vi "S4GUI.vi"(7 "Tab ObsEng":enum32{"Obs", "CCD modes", "Eng"}(tab)) -> ()   [LabVIEW 2018] (continued)
            n1626 = call-dynamic "Read Channel.vi"("error in (no error)"=w3103, "Acquisition in"=w3105) -> ("error out"=w3098:errorcluster, "Channel.lvclass"=w3100:refnum<class "Channel.lvclass">, "Acquisition out"=w3104:refnum<class "Acquisition.lvclass">)  [unwired: 7 in]
            n1627 = call "Write section_name.vi"("error in (no error)"=w3098, "section_name"="CCD_ACS1", "Channel in"=w3100) -> ("error out"=w3097:errorcluster, "Channel out"=w3099:refnum<class "Channel.lvclass">)  [unwired: 7 in]
            n1628 = call-dynamic "save config.vi"("error in (no error)"=w3097, "file config"=w3051, "Channel in"=w3099) -> ("error out"=w3049:errorcluster, "Channel out"=w3050:refnum<class "Channel.lvclass">)  [unwired: 7 in]
            n1629 = call-dynamic "Write Channel.vi"("error in (no error)"=w3049, "Channel.lvclass"=w3050, "Acquisition in"=w3104) -> ("error out"=w3102:errorcluster, "Acquisition out"=w3101:refnum<class "Acquisition.lvclass">)  [unwired: 7 in]
            n1630 = call-dynamic "Write AcquisitionA.vi"("error in (no error)"=w3102, "Acquisition.lvclass"=w3101, "S4ACS_GUI in"=w3106) -> ("error out"=w3062:errorcluster, "S4ACS_GUI out"=w3061:refnum<class "S4GUI.lvclass">)  [unwired: 7 in]
            n1631 = call "Read AcquisitionB.vi"("error in (no error)"=w3062, "S4ACS_GUI in"=w3061) -> ("error out"=w3088:errorcluster, "Acquisition.lvclass"=w3086:refnum<class "Acquisition.lvclass">, "S4ACS_GUI out"=w3085:refnum<class "S4GUI.lvclass">)  [unwired: 7 in]
            n1632 = call-dynamic "Read Channel.vi"("error in (no error)"=w3088, "Acquisition in"=w3086) -> ("error out"=w3093:errorcluster, "Channel.lvclass"=w3091:refnum<class "Channel.lvclass">, "Acquisition out"=w3087:refnum<class "Acquisition.lvclass">)  [unwired: 7 in]
            n1633 = call "Write section_name.vi"("error in (no error)"=w3093, "section_name"="CCD_ACS2", "Channel in"=w3091) -> ("error out"=w3094:errorcluster, "Channel out"=w3092:refnum<class "Channel.lvclass">)  [unwired: 7 in]
            n1634 = call-dynamic "save config.vi"("error in (no error)"=w3094, "file config"=w3051, "Channel in"=w3092) -> ("error out"=w3043:errorcluster, "Channel out"=w3044:refnum<class "Channel.lvclass">)  [unwired: 7 in]
            n1635 = call-dynamic "Write Channel.vi"("error in (no error)"=w3043, "Channel.lvclass"=w3044, "Acquisition in"=w3087) -> ("error out"=w3089:errorcluster, "Acquisition out"=w3090:refnum<class "Acquisition.lvclass">)  [unwired: 7 in]
            n1636 = call "Write AcquisitionB.vi"("error in (no error)"=w3089, "Acquisition.lvclass"=w3090, "S4ACS_GUI in"=w3085) -> ("error out"=w3060:errorcluster, "S4ACS_GUI out"=w3059:refnum<class "S4GUI.lvclass">)  [unwired: 7 in]
            n1637 = call-dynamic "Read AcquisitionC.vi"("error in (no error)"=w3060, "S4ACS_GUI in"=w3059) -> ("error out"=w3081:errorcluster, "Acquisition.lvclass"=w3083:refnum<class "Acquisition.lvclass">, "S4ACS_GUI out"=w3084:refnum<class "S4GUI.lvclass">)  [unwired: 7 in]
            n1638 = call-dynamic "Read Channel.vi"("error in (no error)"=w3081, "Acquisition in"=w3083) -> ("error out"=w3076:errorcluster, "Channel.lvclass"=w3078:refnum<class "Channel.lvclass">, "Acquisition out"=w3082:refnum<class "Acquisition.lvclass">)  [unwired: 7 in]
            n1639 = call "Write section_name.vi"("error in (no error)"=w3076, "section_name"="CCD_ACS3", "Channel in"=w3078) -> ("error out"=w3075:errorcluster, "Channel out"=w3077:refnum<class "Channel.lvclass">)  [unwired: 7 in]
            n1640 = call-dynamic "save config.vi"("error in (no error)"=w3075, "file config"=w3051, "Channel in"=w3077) -> ("error out"=w3045:errorcluster, "Channel out"=w3046:refnum<class "Channel.lvclass">)  [unwired: 7 in]
            n1641 = call-dynamic "Write Channel.vi"("error in (no error)"=w3045, "Channel.lvclass"=w3046, "Acquisition in"=w3082) -> ("error out"=w3080:errorcluster, "Acquisition out"=w3079:refnum<class "Acquisition.lvclass">)  [unwired: 7 in]
            n1642 = call-dynamic "Write AcquisitionC.vi"("error in (no error)"=w3080, "Acquisition.lvclass"=w3079, "S4ACS_GUI in"=w3084) -> ("error out"=w3058:errorcluster, "S4ACS_GUI out"=w3057:refnum<class "S4GUI.lvclass">)  [unwired: 7 in]
            n1643 = call-dynamic "Read AcquisitionD.vi"("error in (no error)"=w3058, "S4ACS_GUI in"=w3057) -> ("error out"=w3066:errorcluster, "Acquisition.lvclass"=w3064:refnum<class "Acquisition.lvclass">, "S4ACS_GUI out"=w3063:refnum<class "S4GUI.lvclass">)  [unwired: 7 in]
            n1644 = call-dynamic "Read Channel.vi"("error in (no error)"=w3066, "Acquisition in"=w3064) -> ("error out"=w3071:errorcluster, "Channel.lvclass"=w3069:refnum<class "Channel.lvclass">, "Acquisition out"=w3065:refnum<class "Acquisition.lvclass">)  [unwired: 7 in]
            n1645 = call "Write section_name.vi"("error in (no error)"=w3071, "section_name"="CCD_ACS4", "Channel in"=w3069) -> ("error out"=w3072:errorcluster, "Channel out"=w3070:refnum<class "Channel.lvclass">)  [unwired: 7 in]
            n1646 = call-dynamic "save config.vi"("error in (no error)"=w3072, "file config"=w3051, "Channel in"=w3070) -> ("error out"=w3047:errorcluster, "Channel out"=w3048:refnum<class "Channel.lvclass">)  [unwired: 7 in]
            n1647 = call-dynamic "Write Channel.vi"("error in (no error)"=w3047, "Channel.lvclass"=w3048, "Acquisition in"=w3065) -> ("error out"=w3067:errorcluster, "Acquisition out"=w3068:refnum<class "Acquisition.lvclass">)  [unwired: 7 in]
            n1648 = call-dynamic "Write AcquisitionD.vi"("error in (no error)"=w3067, "Acquisition.lvclass"=w3068, "S4ACS_GUI in"=w3063) -> ("error out"=w3054:errorcluster, "S4ACS_GUI out"=w3056:refnum<class "S4GUI.lvclass">)  [unwired: 7 in]
            n1649 = call "Write cfg file.vi"("error in (no error)"=w3054, "cfg file"=w3051, "S4ACS_GUI in"=w3056) -> ("error out"=w3053:errorcluster, "S4ACS_GUI out"=w3055:refnum<class "S4GUI.lvclass">)  [unwired: 7 in]
          }
          frame True {
          }
        }
      }
      event "Load Default Button": Value Change {
        w3130 = "default.cfg" ("cfg file name")
        n1650 = event-data() -> ()  [unwired: 1 in, 6 out]
        n1651 = call-dynamic "Read AcquisitionA.vi"("error in (no error)"=w3220, "S4ACS_GUI in"=w3221) -> ("error out"=w3216:errorcluster, "Acquisition.lvclass"=w3218:refnum<class "Acquisition.lvclass">, "S4ACS_GUI out"=w3219:refnum<class "S4GUI.lvclass">)  [unwired: 7 in]
        n1652 = call-dynamic "Read Channel.vi"("error in (no error)"=w3216, "Acquisition in"=w3218) -> ("error out"=w3203:errorcluster, "Channel.lvclass"=w3205:refnum<class "Channel.lvclass">, "Acquisition out"=w3217:refnum<class "Acquisition.lvclass">)  [unwired: 7 in]
        n1653 = call "Write section_name.vi"("error in (no error)"=w3203, "section_name"="CCD_ACS1", "Channel in"=w3205) -> ("error out"=w3202:errorcluster, "Channel out"=w3204:refnum<class "Channel.lvclass">)  [unwired: 7 in]
        n1654 = call-dynamic "load config.vi"("error in (no error)"=w3202, "cfg file name"=w3130, "Channel in"=w3204) -> ("error out"=w3127:errorcluster, "Channel out"=w3129:refnum<class "Channel.lvclass">)  [unwired: 7 in]
        n1655 = call-dynamic "save config.vi"("error in (no error)"=w3127, "file config"="lastsaved.cfg", "Channel in"=w3129) -> ("error out"=w3126:errorcluster, "Channel out"=w3128:refnum<class "Channel.lvclass">)  [unwired: 7 in]
        n1656 = call-dynamic "Read State Machine.vi"("error in (no error)"=w3126, "Device in"=w3128) -> ("error out"=w3212:errorcluster, "State Machine.lvclass"=w3214:refnum<class "State Machine.lvclass">, "Device out"=w3215:refnum<class "Channel.lvclass">)  [unwired: 7 in]
        n1657 = call-dynamic "Write State.vi"("error in (no error)"=w3212, "State"=60, "State Machine in"=w3214) -> ("error out"=w3211:errorcluster, "State Machine out"=w3213:refnum<class "State Machine.lvclass">)  [unwired: 7 in]
        n1658 = call-dynamic "Write State Machine.vi"("error in (no error)"=w3211, "State Machine.lvclass"=w3213, "Device in"=w3215) -> ("error out"=w3208:errorcluster, "Device out"=w3209:refnum<class "Channel.lvclass">)  [unwired: 7 in]
        n1659 = call-dynamic "Write Channel.vi"("error in (no error)"=w3208, "Channel.lvclass"=w3209, "Acquisition in"=w3217) -> ("error out"=w3207:errorcluster, "Acquisition out"=w3206:refnum<class "Acquisition.lvclass">)  [unwired: 7 in]
        n1660 = call-dynamic "Write AcquisitionA.vi"("error in (no error)"=w3207, "Acquisition.lvclass"=w3206, "S4ACS_GUI in"=w3219) -> ("error out"=w3140:errorcluster, "S4ACS_GUI out"=w3139:refnum<class "S4GUI.lvclass">)  [unwired: 7 in]
        n1661 = call "Read AcquisitionB.vi"("error in (no error)"=w3140, "S4ACS_GUI in"=w3139) -> ("error out"=w3184:errorcluster, "Acquisition.lvclass"=w3182:refnum<class "Acquisition.lvclass">, "S4ACS_GUI out"=w3181:refnum<class "S4GUI.lvclass">)  [unwired: 7 in]
        n1662 = call-dynamic "Read Channel.vi"("error in (no error)"=w3184, "Acquisition in"=w3182) -> ("error out"=w3198:errorcluster, "Channel.lvclass"=w3196:refnum<class "Channel.lvclass">, "Acquisition out"=w3183:refnum<class "Acquisition.lvclass">)  [unwired: 7 in]
        n1663 = call "Write section_name.vi"("error in (no error)"=w3198, "section_name"="CCD_ACS2", "Channel in"=w3196) -> ("error out"=w3199:errorcluster, "Channel out"=w3197:refnum<class "Channel.lvclass">)  [unwired: 7 in]
        n1664 = call-dynamic "load config.vi"("error in (no error)"=w3199, "cfg file name"="default.cfg", "Channel in"=w3197) -> ("error out"=w3123:errorcluster, "Channel out"=w3121:refnum<class "Channel.lvclass">)  [unwired: 7 in]
        n1665 = call-dynamic "save config.vi"("error in (no error)"=w3123, "file config"="lastsaved.cfg", "Channel in"=w3121) -> ("error out"=w3122:errorcluster, "Channel out"=w3120:refnum<class "Channel.lvclass">)  [unwired: 7 in]
        n1666 = call-dynamic "Read State Machine.vi"("error in (no error)"=w3122, "Device in"=w3120) -> ("error out"=w3188:errorcluster, "State Machine.lvclass"=w3186:refnum<class "State Machine.lvclass">, "Device out"=w3185:refnum<class "Channel.lvclass">)  [unwired: 7 in]
        n1667 = call-dynamic "Write State.vi"("error in (no error)"=w3188, "State"=60, "State Machine in"=w3186) -> ("error out"=w3189:errorcluster, "State Machine out"=w3187:refnum<class "State Machine.lvclass">)  [unwired: 7 in]
        n1668 = call-dynamic "Write State Machine.vi"("error in (no error)"=w3189, "State Machine.lvclass"=w3187, "Device in"=w3185) -> ("error out"=w3192:errorcluster, "Device out"=w3191:refnum<class "Channel.lvclass">)  [unwired: 7 in]
        n1669 = call-dynamic "Write Channel.vi"("error in (no error)"=w3192, "Channel.lvclass"=w3191, "Acquisition in"=w3183) -> ("error out"=w3193:errorcluster, "Acquisition out"=w3194:refnum<class "Acquisition.lvclass">)  [unwired: 7 in]
        n1670 = call "Write AcquisitionB.vi"("error in (no error)"=w3193, "Acquisition.lvclass"=w3194, "S4ACS_GUI in"=w3181) -> ("error out"=w3138:errorcluster, "S4ACS_GUI out"=w3137:refnum<class "S4GUI.lvclass">)  [unwired: 7 in]
        n1671 = call-dynamic "Read AcquisitionC.vi"("error in (no error)"=w3138, "S4ACS_GUI in"=w3137) -> ("error out"=w3177:errorcluster, "Acquisition.lvclass"=w3179:refnum<class "Acquisition.lvclass">, "S4ACS_GUI out"=w3180:refnum<class "S4GUI.lvclass">)  [unwired: 7 in]
        n1672 = call-dynamic "Read Channel.vi"("error in (no error)"=w3177, "Acquisition in"=w3179) -> ("error out"=w3163:errorcluster, "Channel.lvclass"=w3165:refnum<class "Channel.lvclass">, "Acquisition out"=w3178:refnum<class "Acquisition.lvclass">)  [unwired: 7 in]
        n1673 = call "Write section_name.vi"("error in (no error)"=w3163, "section_name"="CCD_ACS3", "Channel in"=w3165) -> ("error out"=w3162:errorcluster, "Channel out"=w3164:refnum<class "Channel.lvclass">)  [unwired: 7 in]
        n1674 = call-dynamic "load config.vi"("error in (no error)"=w3162, "cfg file name"="default.cfg", "Channel in"=w3164) -> ("error out"=w3117:errorcluster, "Channel out"=w3118:refnum<class "Channel.lvclass">)  [unwired: 7 in]
        n1675 = call-dynamic "save config.vi"("error in (no error)"=w3117, "file config"="lastsaved.cfg", "Channel in"=w3118) -> ("error out"=w3115:errorcluster, "Channel out"=w3116:refnum<class "Channel.lvclass">)  [unwired: 7 in]
        n1676 = call-dynamic "Read State Machine.vi"("error in (no error)"=w3115, "Device in"=w3116) -> ("error out"=w3173:errorcluster, "State Machine.lvclass"=w3175:refnum<class "State Machine.lvclass">, "Device out"=w3176:refnum<class "Channel.lvclass">)  [unwired: 7 in]
        n1677 = call-dynamic "Write State.vi"("error in (no error)"=w3173, "State"=60, "State Machine in"=w3175) -> ("error out"=w3172:errorcluster, "State Machine out"=w3174:refnum<class "State Machine.lvclass">)  [unwired: 7 in]
        n1678 = call-dynamic "Write State Machine.vi"("error in (no error)"=w3172, "State Machine.lvclass"=w3174, "Device in"=w3176) -> ("error out"=w3169:errorcluster, "Device out"=w3170:refnum<class "Channel.lvclass">)  [unwired: 7 in]
        n1679 = call-dynamic "Write Channel.vi"("error in (no error)"=w3169, "Channel.lvclass"=w3170, "Acquisition in"=w3178) -> ("error out"=w3168:errorcluster, "Acquisition out"=w3167:refnum<class "Acquisition.lvclass">)  [unwired: 7 in]
        n1680 = call-dynamic "Write AcquisitionC.vi"("error in (no error)"=w3168, "Acquisition.lvclass"=w3167, "S4ACS_GUI in"=w3180) -> ("error out"=w3136:errorcluster, "S4ACS_GUI out"=w3135:refnum<class "S4GUI.lvclass">)  [unwired: 7 in]
        n1681 = call-dynamic "Read AcquisitionD.vi"("error in (no error)"=w3136, "S4ACS_GUI in"=w3135) -> ("error out"=w3144:errorcluster, "Acquisition.lvclass"=w3142:refnum<class "Acquisition.lvclass">, "S4ACS_GUI out"=w3141:refnum<class "S4GUI.lvclass">)  [unwired: 7 in]
        n1682 = call-dynamic "Read Channel.vi"("error in (no error)"=w3144, "Acquisition in"=w3142) -> ("error out"=w3158:errorcluster, "Channel.lvclass"=w3156:refnum<class "Channel.lvclass">, "Acquisition out"=w3143:refnum<class "Acquisition.lvclass">)  [unwired: 7 in]
        n1683 = call "Write section_name.vi"("error in (no error)"=w3158, "section_name"="CCD_ACS4", "Channel in"=w3156) -> ("error out"=w3159:errorcluster, "Channel out"=w3157:refnum<class "Channel.lvclass">)  [unwired: 7 in]
        n1684 = call-dynamic "load config.vi"("error in (no error)"=w3159, "cfg file name"="default.cfg", "Channel in"=w3157) -> ("error out"=w3113:errorcluster, "Channel out"=w3112:refnum<class "Channel.lvclass">)  [unwired: 7 in]
        n1685 = call-dynamic "save config.vi"("error in (no error)"=w3113, "file config"="lastsaved.cfg", "Channel in"=w3112) -> ("error out"=w3110:errorcluster, "Channel out"=w3111:refnum<class "Channel.lvclass">)  [unwired: 7 in]
        n1686 = call-dynamic "Read State Machine.vi"("error in (no error)"=w3110, "Device in"=w3111) -> ("error out"=w3148:errorcluster, "State Machine.lvclass"=w3146:refnum<class "State Machine.lvclass">, "Device out"=w3145:refnum<class "Channel.lvclass">)  [unwired: 7 in]
        n1687 = call-dynamic "Write State.vi"("error in (no error)"=w3148, "State"=60, "State Machine in"=w3146) -> ("error out"=w3149:errorcluster, "State Machine out"=w3147:refnum<class "State Machine.lvclass">)  [unwired: 7 in]
        n1688 = call-dynamic "Write State Machine.vi"("error in (no error)"=w3149, "State Machine.lvclass"=w3147, "Device in"=w3145) -> ("error out"=w3152:errorcluster, "Device out"=w3151:refnum<class "Channel.lvclass">)  [unwired: 7 in]
        n1689 = call-dynamic "Write Channel.vi"("error in (no error)"=w3152, "Channel.lvclass"=w3151, "Acquisition in"=w3143) -> ("error out"=w3153:errorcluster, "Acquisition out"=w3154:refnum<class "Acquisition.lvclass">)  [unwired: 7 in]
        n1690 = call-dynamic "Write AcquisitionD.vi"("error in (no error)"=w3153, "Acquisition.lvclass"=w3154, "S4ACS_GUI in"=w3141) -> ("error out"=w3132:errorcluster, "S4ACS_GUI out"=w3134:refnum<class "S4GUI.lvclass">)  [unwired: 7 in]
        n1691 = call "Write cfg file.vi"("error in (no error)"=w3132, "cfg file"=w3130, "S4ACS_GUI in"=w3134) -> ("error out"=w3131:errorcluster, "S4ACS_GUI out"=w3133:refnum<class "S4GUI.lvclass">)  [unwired: 7 in]
      }
      event "Restore Default ch2": Value Change {
        n1692 = event-data() -> ()  [unwired: 1 in, 6 out]
        n1693 = call "Read AcquisitionB.vi"("error in (no error)"=w3252, "S4ACS_GUI in"=w3253) -> ("error out"=w3248:errorcluster, "Acquisition.lvclass"=w3250:refnum<class "Acquisition.lvclass">, "S4ACS_GUI out"=w3251:refnum<class "S4GUI.lvclass">)  [unwired: 7 in]
        n1694 = call-dynamic "Read Channel.vi"("error in (no error)"=w3248, "Acquisition in"=w3250) -> ("error out"=w3235:errorcluster, "Channel.lvclass"=w3237:refnum<class "Channel.lvclass">, "Acquisition out"=w3249:refnum<class "Acquisition.lvclass">)  [unwired: 7 in]
        n1695 = call "Write section_name.vi"("error in (no error)"=w3235, "section_name"="CCD_ACS2", "Channel in"=w3237) -> ("error out"=w3234:errorcluster, "Channel out"=w3236:refnum<class "Channel.lvclass">)  [unwired: 7 in]
        n1696 = call-dynamic "load config.vi"("error in (no error)"=w3234, "cfg file name"="default.cfg", "Channel in"=w3236) -> ("error out"=w3232:errorcluster, "Channel out"=w3233:refnum<class "Channel.lvclass">)  [unwired: 7 in]
        n1697 = call-dynamic "Read State Machine.vi"("error in (no error)"=w3232, "Device in"=w3233) -> ("error out"=w3244:errorcluster, "State Machine.lvclass"=w3246:refnum<class "State Machine.lvclass">, "Device out"=w3247:refnum<class "Channel.lvclass">)  [unwired: 7 in]
        n1698 = call-dynamic "Write State.vi"("error in (no error)"=w3244, "State"=60, "State Machine in"=w3246) -> ("error out"=w3243:errorcluster, "State Machine out"=w3245:refnum<class "State Machine.lvclass">)  [unwired: 7 in]
        n1699 = call-dynamic "Write State Machine.vi"("error in (no error)"=w3243, "State Machine.lvclass"=w3245, "Device in"=w3247) -> ("error out"=w3228:errorcluster, "Device out"=w3225:refnum<class "Channel.lvclass">)  [unwired: 7 in]
        n1700 = call "Write section_name.vi"("error in (no error)"=w3228, "section_name"="CCD_ACS2", "Channel in"=w3225) -> ("error out"=w3229:errorcluster, "Channel out"=w3224:refnum<class "Channel.lvclass">)  [unwired: 7 in]
        n1701 = call-dynamic "save config.vi"("error in (no error)"=w3229, "file config"="lastsaved.cfg", "Channel in"=w3224) -> ("error out"=w3227:errorcluster, "Channel out"=w3223:refnum<class "Channel.lvclass">)  [unwired: 7 in]
        n1702 = call-dynamic "Write Channel.vi"("error in (no error)"=w3227, "Channel.lvclass"=w3223, "Acquisition in"=w3249) -> ("error out"=w3241:errorcluster, "Acquisition out"=w3240:refnum<class "Acquisition.lvclass">)  [unwired: 7 in]
        n1703 = call "Write AcquisitionB.vi"("error in (no error)"=w3241, "Acquisition.lvclass"=w3240, "S4ACS_GUI in"=w3251) -> ("error out"=w3239:errorcluster, "S4ACS_GUI out"=w3230:refnum<class "S4GUI.lvclass">)  [unwired: 7 in]
      }
      event "Restore Default ch3": Value Change {
        n1704 = event-data() -> ()  [unwired: 1 in, 6 out]
        n1705 = call-dynamic "Read AcquisitionC.vi"("error in (no error)"=w3284, "S4ACS_GUI in"=w3285) -> ("error out"=w3280:errorcluster, "Acquisition.lvclass"=w3282:refnum<class "Acquisition.lvclass">, "S4ACS_GUI out"=w3283:refnum<class "S4GUI.lvclass">)  [unwired: 7 in]
        n1706 = call-dynamic "Read Channel.vi"("error in (no error)"=w3280, "Acquisition in"=w3282) -> ("error out"=w3267:errorcluster, "Channel.lvclass"=w3269:refnum<class "Channel.lvclass">, "Acquisition out"=w3281:refnum<class "Acquisition.lvclass">)  [unwired: 7 in]
        n1707 = call "Write section_name.vi"("error in (no error)"=w3267, "section_name"="CCD_ACS3", "Channel in"=w3269) -> ("error out"=w3266:errorcluster, "Channel out"=w3268:refnum<class "Channel.lvclass">)  [unwired: 7 in]
        n1708 = call-dynamic "load config.vi"("error in (no error)"=w3266, "cfg file name"="default.cfg", "Channel in"=w3268) -> ("error out"=w3264:errorcluster, "Channel out"=w3265:refnum<class "Channel.lvclass">)  [unwired: 7 in]
        n1709 = call-dynamic "Read State Machine.vi"("error in (no error)"=w3264, "Device in"=w3265) -> ("error out"=w3276:errorcluster, "State Machine.lvclass"=w3278:refnum<class "State Machine.lvclass">, "Device out"=w3279:refnum<class "Channel.lvclass">)  [unwired: 7 in]
        n1710 = call-dynamic "Write State.vi"("error in (no error)"=w3276, "State"=60, "State Machine in"=w3278) -> ("error out"=w3275:errorcluster, "State Machine out"=w3277:refnum<class "State Machine.lvclass">)  [unwired: 7 in]
        n1711 = call-dynamic "Write State Machine.vi"("error in (no error)"=w3275, "State Machine.lvclass"=w3277, "Device in"=w3279) -> ("error out"=w3255:errorcluster, "Device out"=w3257:refnum<class "Channel.lvclass">)  [unwired: 7 in]
        n1712 = call "Write section_name.vi"("error in (no error)"=w3255, "section_name"="CCD_ACS3", "Channel in"=w3257) -> ("error out"=w3261:errorcluster, "Channel out"=w3256:refnum<class "Channel.lvclass">)  [unwired: 7 in]
        n1713 = call-dynamic "save config.vi"("error in (no error)"=w3261, "file config"="lastsaved.cfg", "Channel in"=w3256) -> ("error out"=w3254:errorcluster, "Channel out"=w3258:refnum<class "Channel.lvclass">)  [unwired: 7 in]
        n1714 = call-dynamic "Write Channel.vi"("error in (no error)"=w3254, "Channel.lvclass"=w3258, "Acquisition in"=w3281) -> ("error out"=w3273:errorcluster, "Acquisition out"=w3272:refnum<class "Acquisition.lvclass">)  [unwired: 7 in]
        n1715 = call-dynamic "Write AcquisitionC.vi"("error in (no error)"=w3273, "Acquisition.lvclass"=w3272, "S4ACS_GUI in"=w3283) -> ("error out"=w3271:errorcluster, "S4ACS_GUI out"=w3262:refnum<class "S4GUI.lvclass">)  [unwired: 7 in]
      }
      event "Restore Default ch4": Value Change {
        n1716 = event-data() -> ()  [unwired: 1 in, 6 out]
        n1717 = call-dynamic "Read AcquisitionD.vi"("error in (no error)"=w3316, "S4ACS_GUI in"=w3317) -> ("error out"=w3312:errorcluster, "Acquisition.lvclass"=w3314:refnum<class "Acquisition.lvclass">, "S4ACS_GUI out"=w3315:refnum<class "S4GUI.lvclass">)  [unwired: 7 in]
        n1718 = call-dynamic "Read Channel.vi"("error in (no error)"=w3312, "Acquisition in"=w3314) -> ("error out"=w3299:errorcluster, "Channel.lvclass"=w3301:refnum<class "Channel.lvclass">, "Acquisition out"=w3313:refnum<class "Acquisition.lvclass">)  [unwired: 7 in]
        n1719 = call "Write section_name.vi"("error in (no error)"=w3299, "section_name"="CCD_ACS4", "Channel in"=w3301) -> ("error out"=w3298:errorcluster, "Channel out"=w3300:refnum<class "Channel.lvclass">)  [unwired: 7 in]
        n1720 = call-dynamic "load config.vi"("error in (no error)"=w3298, "cfg file name"="default.cfg", "Channel in"=w3300) -> ("error out"=w3296:errorcluster, "Channel out"=w3297:refnum<class "Channel.lvclass">)  [unwired: 7 in]
        n1721 = call-dynamic "Read State Machine.vi"("error in (no error)"=w3296, "Device in"=w3297) -> ("error out"=w3308:errorcluster, "State Machine.lvclass"=w3310:refnum<class "State Machine.lvclass">, "Device out"=w3311:refnum<class "Channel.lvclass">)  [unwired: 7 in]
        n1722 = call-dynamic "Write State.vi"("error in (no error)"=w3308, "State"=60, "State Machine in"=w3310) -> ("error out"=w3307:errorcluster, "State Machine out"=w3309:refnum<class "State Machine.lvclass">)  [unwired: 7 in]
        n1723 = call-dynamic "Write State Machine.vi"("error in (no error)"=w3307, "State Machine.lvclass"=w3309, "Device in"=w3311) -> ("error out"=w3287:errorcluster, "Device out"=w3290:refnum<class "Channel.lvclass">)  [unwired: 7 in]
        n1724 = call "Write section_name.vi"("error in (no error)"=w3287, "section_name"="CCD_ACS4", "Channel in"=w3290) -> ("error out"=w3293:errorcluster, "Channel out"=w3289:refnum<class "Channel.lvclass">)  [unwired: 7 in]
        n1725 = call-dynamic "save config.vi"("error in (no error)"=w3293, "file config"="lastsaved.cfg", "Channel in"=w3289) -> ("error out"=w3286:errorcluster, "Channel out"=w3288:refnum<class "Channel.lvclass">)  [unwired: 7 in]
        n1726 = call-dynamic "Write Channel.vi"("error in (no error)"=w3286, "Channel.lvclass"=w3288, "Acquisition in"=w3313) -> ("error out"=w3305:errorcluster, "Acquisition out"=w3304:refnum<class "Acquisition.lvclass">)  [unwired: 7 in]
        n1727 = call-dynamic "Write AcquisitionD.vi"("error in (no error)"=w3305, "Acquisition.lvclass"=w3304, "S4ACS_GUI in"=w3315) -> ("error out"=w3303:errorcluster, "S4ACS_GUI out"=w3294:refnum<class "S4GUI.lvclass">)  [unwired: 7 in]
      }
      event "Copy to Input ch1": Value Change {
        w3318 = T12."Enabled" ("Disabled")
        n1728 = event-data() -> ()  [unwired: 1 in, 6 out]
        n1729 = call-dynamic "Read AcquisitionA.vi"("error in (no error)"=w3351, "S4ACS_GUI in"=w3352) -> ("error out"=w3347:errorcluster, "Acquisition.lvclass"=w3350:refnum<class "Acquisition.lvclass">, "S4ACS_GUI out"=w3319:refnum<class "S4GUI.lvclass">)  [unwired: 7 in]
        n1730 = call-dynamic "Read Channel.vi"("error in (no error)"=w3347, "Acquisition in"=w3350) -> ("error out"=w3346:errorcluster, "Channel.lvclass"=w3349:refnum<class "Channel.lvclass">)  [unwired: 7 in, 1 out]
        n1731 = call-dynamic "Read Interface.vi"("error in (no error)"=w3346, "Channel in"=w3349) -> ("error out"=w3345:errorcluster, "Interface.lvclass"=w3348:refnum<class "Interface.lvclass">)  [unwired: 7 in, 1 out]
        n1732 = call-dynamic "Get CCD_Config.vi"("error in (no error)"=w3345, "Interface in"=w3348) -> ("error out"=w3342:errorcluster, "output cluster"=w3341:T30)  [unwired: 7 in, 1 out]
        n1733 = Unbundle By Name(w3341) -> ("INITIAL_LINE"=w3340:u16, "INITIAL_COLUMN"=w3339:u16, "FINAL_LINE"=w3338:u16, "FINAL_COLUMN"=w3337:u16, "VBIN"=w3336:u16, "HBIN"=w3335:u16, "PREAMP"=w3334:u8, "EM_GAIN"=w3333:u16, "READOUT_RATE"=w3332:u8, "SHUTTER_OPENING_TIME"=w3331:u16, "SHUTTER_CLOSING_TIME"=w3330:u16, "VERTICAL_SHIFT_SPEED"=w3329:u8, "READ_MODE"=w3328:u8, "VERTICAL_CLOCK_VOLTAGE"=w3327:u8, "AD_CHANNEL"=w3326:u32, "SHUTTER_MODE"=w3325:u8, "SHUTTER_TTL"=w3324:u8, "TRIGGER_MODE"=w3323:u8, "FRAME_TRANSFER"=w3322:bool, "ACQUISITION_MODE"=w3321:u8, "EM_MODE"=w3320:u8)
        n1734 = local read "Input Cluster"() -> (w3344:T8)
        n1735 = Bundle By Name(cluster=w3344, "Parameters.Image \nInitial Line"=w3340, "Parameters.Image\nInitial Column"=w3339, "Parameters.Image\nFinal Line"=w3338, "Parameters.Image\nFInal Column"=w3337, "Parameters.Vertical\nBinning"=w3336, "Parameters.Horizontal\nBinning"=w3335, "Parameters.Pre-amplification\nGain"=w3334, "Parameters.CCD\nEM Gain"=w3333, "Parameters.Readout\nRate"=w3332, "Parameters.Shutter\nOpenning Time"=w3331, "Parameters.Shutter\nClosing Time"=w3330, "Parameters.Vertical\nShift Speed"=w3329, "Parameters.Read\nMode"=w3328, "Parameters.Vertical\nClock Voltage"=w3327, "Parameters.A/D \nChannel"=w3326, "Parameters.Shutter\nMode"=w3325, "Parameters.Shutter\nTTL"=w3324, "Parameters.Trigger\nMode"=w3323, "Parameters.Frame\nTransfer"=w3322, "Parameters.Acquisition\nMode"=w3321, "Parameters.CCD \nEM Mode"=w3320) -> (w3343:T8)
        n1736 = local write "Input Cluster"(w3343) -> ()
        n1737 = property on="Set from Input ch1" class="Bool"("DisabledEnum"=w3318) -> ()  [unwired: 2 in, 2 out]
        n1738 = property on="Set from Input ch3" class="Bool"("DisabledEnum"=w3318) -> ()  [unwired: 2 in, 2 out]
        n1739 = property on="Set from Input ch2" class="Bool"("DisabledEnum"=w3318) -> ()  [unwired: 2 in, 2 out]
        n1740 = property on="Set from Input ch4" class="Bool"("DisabledEnum"=w3318) -> ()  [unwired: 2 in, 2 out]
      }
      event "Copy to Input ch2": Value Change {
        w3353 = T12."Enabled" ("Disabled")
        n1741 = event-data() -> ()  [unwired: 1 in, 6 out]
        n1742 = call "Read AcquisitionB.vi"("error in (no error)"=w3386, "S4ACS_GUI in"=w3387) -> ("error out"=w3382:errorcluster, "Acquisition.lvclass"=w3385:refnum<class "Acquisition.lvclass">, "S4ACS_GUI out"=w3354:refnum<class "S4GUI.lvclass">)  [unwired: 7 in]
        n1743 = call-dynamic "Read Channel.vi"("error in (no error)"=w3382, "Acquisition in"=w3385) -> ("error out"=w3381:errorcluster, "Channel.lvclass"=w3384:refnum<class "Channel.lvclass">)  [unwired: 7 in, 1 out]
        n1744 = call-dynamic "Read Interface.vi"("error in (no error)"=w3381, "Channel in"=w3384) -> ("error out"=w3380:errorcluster, "Interface.lvclass"=w3383:refnum<class "Interface.lvclass">)  [unwired: 7 in, 1 out]
        n1745 = call-dynamic "Get CCD_Config.vi"("error in (no error)"=w3380, "Interface in"=w3383) -> ("error out"=w3377:errorcluster, "output cluster"=w3376:T30)  [unwired: 7 in, 1 out]
        n1746 = Unbundle By Name(w3376) -> ("INITIAL_LINE"=w3375:u16, "INITIAL_COLUMN"=w3374:u16, "FINAL_LINE"=w3373:u16, "FINAL_COLUMN"=w3372:u16, "VBIN"=w3371:u16, "HBIN"=w3370:u16, "PREAMP"=w3369:u8, "EM_GAIN"=w3368:u16, "READOUT_RATE"=w3367:u8, "SHUTTER_OPENING_TIME"=w3366:u16, "SHUTTER_CLOSING_TIME"=w3365:u16, "VERTICAL_SHIFT_SPEED"=w3364:u8, "READ_MODE"=w3363:u8, "VERTICAL_CLOCK_VOLTAGE"=w3362:u8, "AD_CHANNEL"=w3361:u32, "SHUTTER_MODE"=w3360:u8, "SHUTTER_TTL"=w3359:u8, "TRIGGER_MODE"=w3358:u8, "FRAME_TRANSFER"=w3357:bool, "ACQUISITION_MODE"=w3356:u8, "EM_MODE"=w3355:u8)
        n1747 = local read "Input Cluster"() -> (w3379:T8)
        n1748 = Bundle By Name(cluster=w3379, "Parameters.Image \nInitial Line"=w3375, "Parameters.Image\nInitial Column"=w3374, "Parameters.Image\nFinal Line"=w3373, "Parameters.Image\nFInal Column"=w3372, "Parameters.Vertical\nBinning"=w3371, "Parameters.Horizontal\nBinning"=w3370, "Parameters.Pre-amplification\nGain"=w3369, "Parameters.CCD\nEM Gain"=w3368, "Parameters.Readout\nRate"=w3367, "Parameters.Shutter\nOpenning Time"=w3366, "Parameters.Shutter\nClosing Time"=w3365, "Parameters.Vertical\nShift Speed"=w3364, "Parameters.Read\nMode"=w3363, "Parameters.Vertical\nClock Voltage"=w3362, "Parameters.A/D \nChannel"=w3361, "Parameters.Shutter\nMode"=w3360, "Parameters.Shutter\nTTL"=w3359, "Parameters.Trigger\nMode"=w3358, "Parameters.Frame\nTransfer"=w3357, "Parameters.Acquisition\nMode"=w3356, "Parameters.CCD \nEM Mode"=w3355) -> (w3378:T8)
        n1749 = local write "Input Cluster"(w3378) -> ()
        n1750 = property on="Set from Input ch1" class="Bool"("DisabledEnum"=w3353) -> ()  [unwired: 2 in, 2 out]
        n1751 = property on="Set from Input ch3" class="Bool"("DisabledEnum"=w3353) -> ()  [unwired: 2 in, 2 out]
        n1752 = property on="Set from Input ch2" class="Bool"("DisabledEnum"=w3353) -> ()  [unwired: 2 in, 2 out]
        n1753 = property on="Set from Input ch4" class="Bool"("DisabledEnum"=w3353) -> ()  [unwired: 2 in, 2 out]
      }
      event "Copy to Input ch3": Value Change {
        w3388 = T12."Enabled" ("Disabled")
        n1754 = event-data() -> ()  [unwired: 1 in, 6 out]
        n1755 = call-dynamic "Read AcquisitionC.vi"("error in (no error)"=w3421, "S4ACS_GUI in"=w3422) -> ("error out"=w3417:errorcluster, "Acquisition.lvclass"=w3420:refnum<class "Acquisition.lvclass">, "S4ACS_GUI out"=w3389:refnum<class "S4GUI.lvclass">)  [unwired: 7 in]
        n1756 = call-dynamic "Read Channel.vi"("error in (no error)"=w3417, "Acquisition in"=w3420) -> ("error out"=w3416:errorcluster, "Channel.lvclass"=w3419:refnum<class "Channel.lvclass">)  [unwired: 7 in, 1 out]
        n1757 = call-dynamic "Read Interface.vi"("error in (no error)"=w3416, "Channel in"=w3419) -> ("error out"=w3415:errorcluster, "Interface.lvclass"=w3418:refnum<class "Interface.lvclass">)  [unwired: 7 in, 1 out]
        n1758 = call-dynamic "Get CCD_Config.vi"("error in (no error)"=w3415, "Interface in"=w3418) -> ("error out"=w3412:errorcluster, "output cluster"=w3411:T30)  [unwired: 7 in, 1 out]
        n1759 = Unbundle By Name(w3411) -> ("INITIAL_LINE"=w3410:u16, "INITIAL_COLUMN"=w3409:u16, "FINAL_LINE"=w3408:u16, "FINAL_COLUMN"=w3407:u16, "VBIN"=w3406:u16, "HBIN"=w3405:u16, "PREAMP"=w3404:u8, "EM_GAIN"=w3403:u16, "READOUT_RATE"=w3402:u8, "SHUTTER_OPENING_TIME"=w3401:u16, "SHUTTER_CLOSING_TIME"=w3400:u16, "VERTICAL_SHIFT_SPEED"=w3399:u8, "READ_MODE"=w3398:u8, "VERTICAL_CLOCK_VOLTAGE"=w3397:u8, "AD_CHANNEL"=w3396:u32, "SHUTTER_MODE"=w3395:u8, "SHUTTER_TTL"=w3394:u8, "TRIGGER_MODE"=w3393:u8, "FRAME_TRANSFER"=w3392:bool, "ACQUISITION_MODE"=w3391:u8, "EM_MODE"=w3390:u8)
        n1760 = local read "Input Cluster"() -> (w3414:T8)
        n1761 = Bundle By Name(cluster=w3414, "Parameters.Image \nInitial Line"=w3410, "Parameters.Image\nInitial Column"=w3409, "Parameters.Image\nFinal Line"=w3408, "Parameters.Image\nFInal Column"=w3407, "Parameters.Vertical\nBinning"=w3406, "Parameters.Horizontal\nBinning"=w3405, "Parameters.Pre-amplification\nGain"=w3404, "Parameters.CCD\nEM Gain"=w3403, "Parameters.Readout\nRate"=w3402, "Parameters.Shutter\nOpenning Time"=w3401, "Parameters.Shutter\nClosing Time"=w3400, "Parameters.Vertical\nShift Speed"=w3399, "Parameters.Read\nMode"=w3398, "Parameters.Vertical\nClock Voltage"=w3397, "Parameters.A/D \nChannel"=w3396, "Parameters.Shutter\nMode"=w3395, "Parameters.Shutter\nTTL"=w3394, "Parameters.Trigger\nMode"=w3393, "Parameters.Frame\nTransfer"=w3392, "Parameters.Acquisition\nMode"=w3391, "Parameters.CCD \nEM Mode"=w3390) -> (w3413:T8)
        n1762 = local write "Input Cluster"(w3413) -> ()
        n1763 = property on="Set from Input ch1" class="Bool"("DisabledEnum"=w3388) -> ()  [unwired: 2 in, 2 out]
        n1764 = property on="Set from Input ch3" class="Bool"("DisabledEnum"=w3388) -> ()  [unwired: 2 in, 2 out]
        n1765 = property on="Set from Input ch2" class="Bool"("DisabledEnum"=w3388) -> ()  [unwired: 2 in, 2 out]
        n1766 = property on="Set from Input ch4" class="Bool"("DisabledEnum"=w3388) -> ()  [unwired: 2 in, 2 out]
      }
      event "Copy to Input ch4": Value Change {
        w3423 = T12."Enabled" ("Disabled")
        n1767 = event-data() -> ()  [unwired: 1 in, 6 out]
        n1768 = call-dynamic "Read AcquisitionD.vi"("error in (no error)"=w3456, "S4ACS_GUI in"=w3457) -> ("error out"=w3452:errorcluster, "Acquisition.lvclass"=w3455:refnum<class "Acquisition.lvclass">, "S4ACS_GUI out"=w3424:refnum<class "S4GUI.lvclass">)  [unwired: 7 in]
        n1769 = call-dynamic "Read Channel.vi"("error in (no error)"=w3452, "Acquisition in"=w3455) -> ("error out"=w3451:errorcluster, "Channel.lvclass"=w3454:refnum<class "Channel.lvclass">)  [unwired: 7 in, 1 out]
        n1770 = call-dynamic "Read Interface.vi"("error in (no error)"=w3451, "Channel in"=w3454) -> ("error out"=w3450:errorcluster, "Interface.lvclass"=w3453:refnum<class "Interface.lvclass">)  [unwired: 7 in, 1 out]
        n1771 = call-dynamic "Get CCD_Config.vi"("error in (no error)"=w3450, "Interface in"=w3453) -> ("error out"=w3447:errorcluster, "output cluster"=w3446:T30)  [unwired: 7 in, 1 out]
        n1772 = Unbundle By Name(w3446) -> ("INITIAL_LINE"=w3445:u16, "INITIAL_COLUMN"=w3444:u16, "FINAL_LINE"=w3443:u16, "FINAL_COLUMN"=w3442:u16, "VBIN"=w3441:u16, "HBIN"=w3440:u16, "PREAMP"=w3439:u8, "EM_GAIN"=w3438:u16, "READOUT_RATE"=w3437:u8, "SHUTTER_OPENING_TIME"=w3436:u16, "SHUTTER_CLOSING_TIME"=w3435:u16, "VERTICAL_SHIFT_SPEED"=w3434:u8, "READ_MODE"=w3433:u8, "VERTICAL_CLOCK_VOLTAGE"=w3432:u8, "AD_CHANNEL"=w3431:u32, "SHUTTER_MODE"=w3430:u8, "SHUTTER_TTL"=w3429:u8, "TRIGGER_MODE"=w3428:u8, "FRAME_TRANSFER"=w3427:bool, "ACQUISITION_MODE"=w3426:u8, "EM_MODE"=w3425:u8)
        n1773 = local read "Input Cluster"() -> (w3449:T8)
        n1774 = Bundle By Name(cluster=w3449, "Parameters.Image \nInitial Line"=w3445, "Parameters.Image\nInitial Column"=w3444, "Parameters.Image\nFinal Line"=w3443, "Parameters.Image\nFInal Column"=w3442, "Parameters.Vertical\nBinning"=w3441, "Parameters.Horizontal\nBinning"=w3440, "Parameters.Pre-amplification\nGain"=w3439, "Parameters.CCD\nEM Gain"=w3438, "Parameters.Readout\nRate"=w3437, "Parameters.Shutter\nOpenning Time"=w3436, "Parameters.Shutter\nClosing Time"=w3435, "Parameters.Vertical\nShift Speed"=w3434, "Parameters.Read\nMode"=w3433, "Parameters.Vertical\nClock Voltage"=w3432, "Parameters.A/D \nChannel"=w3431, "Parameters.Shutter\nMode"=w3430, "Parameters.Shutter\nTTL"=w3429, "Parameters.Trigger\nMode"=w3428, "Parameters.Frame\nTransfer"=w3427, "Parameters.Acquisition\nMode"=w3426, "Parameters.CCD \nEM Mode"=w3425) -> (w3448:T8)
        n1775 = local write "Input Cluster"(w3448) -> ()
        n1776 = property on="Set from Input ch1" class="Bool"("DisabledEnum"=w3423) -> ()  [unwired: 2 in, 2 out]
        n1777 = property on="Set from Input ch3" class="Bool"("DisabledEnum"=w3423) -> ()  [unwired: 2 in, 2 out]
        n1778 = property on="Set from Input ch2" class="Bool"("DisabledEnum"=w3423) -> ()  [unwired: 2 in, 2 out]
        n1779 = property on="Set from Input ch4" class="Bool"("DisabledEnum"=w3423) -> ()  [unwired: 2 in, 2 out]
      }
      event "Scrollbar": Value Change {
        (unwired) 765.0 ("BarOffset")
        (unwired) 1000.0 ("BarOffset")
        n1780 = event-data() -> ()  [unwired: 1 in, 6 out]
        n1781 = disable-structure shown="Disabled" {
          disable-tunnel: w3459 -> [w3471 _]
          frame Disabled {
            # "como alterar o valor de um parametro em \"Parameter Input\""
            n1782 = Unbundle By Name(w3471) -> ("Parameters"=w3473:T5)
            n1783 = Bundle By Name(cluster=w3473, "Readout\nRate"=u8 1 ("Readout\nRate")) -> (w3470:T5)
            n1784 = Bundle By Name(cluster=w3471, "Parameters"=w3470) -> (w3469:T8)
            n1785 = local write "Input Cluster"(w3469) -> ()
          }
          frame Enabled {
          }
        }
        n1786 = property on="Scrollbar" class="Scroll (strict)"() -> ("DocMax"=w3463:dbl)  [unwired: 2 in, 2 out]
        n1787 = Unbundle(w3461) -> ("Parameters"=w3466:refnum<vi>, "Current Configuration"=w3465:refnum<vi>)
        n1788 = Subtract(x=w3463, y="Scrollbar") -> (x-y=w3467:dbl)
        n1789 = Subtract(x=w3467, y=200.0 ("BarOffset")) -> (x-y=w3464:dbl)
        n1790 = property on="Property Node" class="Clust (strict)"(reference=w3466, "Top"=w3464) -> ()  [unwired: 1 in, 2 out]
        n1791 = property on="Property Node" class="Clust (strict)"(reference=w3465, "Top"=w3464) -> ()  [unwired: 1 in, 2 out]
      }
      event "Select Positions": Value Change {
        # "Garantir que, quando em POLARIMETRIA, pelo menos WP1 esteja selecionado."
        n1792 = event-data() -> ()  [unwired: 1 in, 6 out]
        n1793 = call "Read Instrument.lvclass.vi"("error in (no error)"=w3495, "S4ACS_GUI in"=w3494) -> ("error out"=w3504:errorcluster, "Instrument.lvclass"=w3503:refnum<class "Instrument.lvclass">, "S4ACS_GUI out"=w3497:refnum<class "S4GUI.lvclass">)  [unwired: 7 in]
        n1794 = call "Read WPROT.vi"("error in (no error)"=w3504, "Instrument in"=w3503) -> ("error out"=w3496:errorcluster, "Opt_Selector.lvclass"=w3500:refnum<class "Opt_Selector.lvclass">, "Instrument out"=w3498:refnum<class "Instrument.lvclass">)  [unwired: 7 in]
        n1795 = case shown="4" "Select Positions" {
          tunnel: w3496 -> [w3538 w3551 w3564 w3577 w3590 w3599]
          tunnel: [w3536 w3549 w3562 w3572 w3588 w3598] -> w3499
          tunnel: [w3533 w3547 w3560 w3574 w3586 w3599] -> w3492
          tunnel: w3500 -> [w3539 w3552 w3565 w3578 w3591 w3598]
          tunnel: [16 8 4 8 0 0] -> w3493
          tunnel: [0.0 ("Scale.Range:Minimum") 0.0 ("Scale.Range:Minimum") 0.0 ("Scale.Range:Minimum") 0.0 ("Scale.Range:Minimum") 0.0 ("Scale.Range:Minimum") 0.0 ("Scale.Range:Minimum")] -> w3491
          frame 0, Default {
            w3535 = u16 65535 ("sequencia")
            w3540 = TRUE ("P0")
            w3541 = TRUE ("P0")
            w3542 = TRUE ("P0")
            w3543 = TRUE ("P0")
            # "1111 1111 1111 1111 = 65.535"
            n1796 = local write "P0"(w3543) -> ()
            n1797 = local write "P1"(w3543) -> ()
            n1798 = local write "P2"(w3543) -> ()
            n1799 = local write "P3"(w3543) -> ()
            n1800 = local write "P4"(w3541) -> ()
            n1801 = local write "P5"(w3541) -> ()
            n1802 = local write "P6"(w3541) -> ()
            n1803 = local write "P7"(w3541) -> ()
            n1804 = call-dynamic "Write sequencia.vi"("error in (no error)"=w3538, "sequencia"=w3535, "Opt_Selector in"=w3539) -> ("error out"=w3534:errorcluster, "Opt_Selector out"=w3537:refnum<class "Opt_Selector.lvclass">)  [unwired: 7 in]
            n1805 = call-dynamic "Write sequencia_ant.vi"("error in (no error)"=w3534, "sequencia_ant"=w3535, "Opt_Selector in"=w3537) -> ("error out"=w3533:errorcluster, "Opt_Selector out"=w3536:refnum<class "Opt_Selector.lvclass">)  [unwired: 7 in]
            n1806 = local write "P8"(w3542) -> ()
            n1807 = local write "P9"(w3542) -> ()
            n1808 = local write "P10"(w3542) -> ()
            n1809 = local write "P11"(w3542) -> ()
            n1810 = local write "P12"(w3540) -> ()
            n1811 = local write "P13"(w3540) -> ()
            n1812 = local write "P14"(w3540) -> ()
            n1813 = local write "P15"(w3540) -> ()
          }
          frame 1 {
            w3546 = u16 255 ("sequencia")
            w3553 = FALSE ("P0")
            w3554 = TRUE ("P0")
            w3555 = FALSE ("P0")
            w3556 = TRUE ("P0")
            # "0000 0000 1111 1111 = 255"
            n1814 = local write "P0"(w3556) -> ()
            n1815 = local write "P1"(w3556) -> ()
            n1816 = local write "P2"(w3556) -> ()
            n1817 = local write "P3"(w3556) -> ()
            n1818 = local write "P4"(w3554) -> ()
            n1819 = local write "P5"(w3554) -> ()
            n1820 = local write "P6"(w3554) -> ()
            n1821 = local write "P7"(w3554) -> ()
            n1822 = call-dynamic "Write sequencia.vi"("error in (no error)"=w3551, "sequencia"=w3546, "Opt_Selector in"=w3552) -> ("error out"=w3548:errorcluster, "Opt_Selector out"=w3550:refnum<class "Opt_Selector.lvclass">)  [unwired: 7 in]
            n1823 = local write "P8"(w3555) -> ()
            n1824 = local write "P9"(w3555) -> ()
            n1825 = local write "P10"(w3555) -> ()
            n1826 = local write "P11"(w3555) -> ()
            n1827 = local write "P12"(w3553) -> ()
            n1828 = local write "P13"(w3553) -> ()
            n1829 = local write "P14"(w3553) -> ()
            n1830 = local write "P15"(w3553) -> ()
            n1831 = call-dynamic "Write sequencia_ant.vi"("error in (no error)"=w3548, "sequencia_ant"=w3546, "Opt_Selector in"=w3550) -> ("error out"=w3547:errorcluster, "Opt_Selector out"=w3549:refnum<class "Opt_Selector.lvclass">)  [unwired: 7 in]
          }
          frame 2 {
            w3559 = u16 15 ("sequencia")
            w3566 = FALSE ("P0")
            w3567 = FALSE ("P0")
            w3568 = FALSE ("P0")
            w3569 = TRUE ("P0")
            # "0000 0000 0000 1111 = 15"
            n1832 = local write "P0"(w3569) -> ()
            n1833 = local write "P1"(w3569) -> ()
            n1834 = local write "P2"(w3569) -> ()
            n1835 = local write "P3"(w3569) -> ()
            n1836 = local write "P4"(w3567) -> ()
            n1837 = local write "P5"(w3567) -> ()
            n1838 = local write "P6"(w3567) -> ()
            n1839 = local write "P7"(w3567) -> ()
            n1840 = call-dynamic "Write sequencia.vi"("error in (no error)"=w3564, "sequencia"=w3559, "Opt_Selector in"=w3565) -> ("error out"=w3561:errorcluster, "Opt_Selector out"=w3563:refnum<class "Opt_Selector.lvclass">)  [unwired: 7 in]
            n1841 = call-dynamic "Write sequencia_ant.vi"("error in (no error)"=w3561, "sequencia_ant"=w3559, "Opt_Selector in"=w3563) -> ("error out"=w3560:errorcluster, "Opt_Selector out"=w3562:refnum<class "Opt_Selector.lvclass">)  [unwired: 7 in]
            n1842 = local write "P8"(w3568) -> ()
            n1843 = local write "P9"(w3568) -> ()
            n1844 = local write "P10"(w3568) -> ()
            n1845 = local write "P11"(w3568) -> ()
            n1846 = local write "P12"(w3566) -> ()
            n1847 = local write "P13"(w3566) -> ()
            n1848 = local write "P14"(w3566) -> ()
            n1849 = local write "P15"(w3566) -> ()
          }
          frame 3 {
            w3573 = u16 3855 ("sequencia")
            w3579 = FALSE ("P0")
            w3580 = FALSE ("P0")
            w3581 = TRUE ("P0")
            w3582 = TRUE ("P0")
            # "0000 1111 0000 1111 = 3855"
            n1850 = local write "P0"(w3582) -> ()
            n1851 = local write "P1"(w3582) -> ()
            n1852 = local write "P2"(w3582) -> ()
            n1853 = local write "P3"(w3582) -> ()
            n1854 = local write "P4"(w3580) -> ()
            n1855 = local write "P5"(w3580) -> ()
            n1856 = local write "P6"(w3580) -> ()
            n1857 = local write "P7"(w3580) -> ()
            n1858 = call-dynamic "Write sequencia.vi"("error in (no error)"=w3577, "sequencia"=w3573, "Opt_Selector in"=w3578) -> ("error out"=w3575:errorcluster, "Opt_Selector out"=w3576:refnum<class "Opt_Selector.lvclass">)  [unwired: 7 in]
            n1859 = local write "P8"(w3581) -> ()
            n1860 = local write "P9"(w3581) -> ()
            n1861 = local write "P10"(w3581) -> ()
            n1862 = local write "P11"(w3581) -> ()
            n1863 = local write "P12"(w3579) -> ()
            n1864 = local write "P13"(w3579) -> ()
            n1865 = local write "P14"(w3579) -> ()
            n1866 = local write "P15"(w3579) -> ()
            n1867 = call-dynamic "Write sequencia_ant.vi"("error in (no error)"=w3575, "sequencia_ant"=w3573, "Opt_Selector in"=w3576) -> ("error out"=w3574:errorcluster, "Opt_Selector out"=w3572:refnum<class "Opt_Selector.lvclass">)  [unwired: 7 in]
          }
          frame 4 {
            w3585 = u16 0 ("sequencia")
            w3592 = FALSE ("P0")
            w3593 = FALSE ("P0")
            w3594 = FALSE ("P0")
            w3595 = FALSE ("P0")
            n1868 = local write "P0"(w3595) -> ()
            n1869 = local write "P1"(w3595) -> ()
            n1870 = local write "P2"(w3595) -> ()
            n1871 = local write "P3"(w3595) -> ()
            n1872 = local write "P4"(w3593) -> ()
            n1873 = local write "P5"(w3593) -> ()
            n1874 = local write "P6"(w3593) -> ()
            n1875 = local write "P7"(w3593) -> ()
            n1876 = call-dynamic "Write sequencia.vi"("error in (no error)"=w3590, "sequencia"=w3585, "Opt_Selector in"=w3591) -> ("error out"=w3587:errorcluster, "Opt_Selector out"=w3589:refnum<class "Opt_Selector.lvclass">)  [unwired: 7 in]
            n1877 = call-dynamic "Write sequencia_ant.vi"("error in (no error)"=w3587, "sequencia_ant"=w3585, "Opt_Selector in"=w3589) -> ("error out"=w3586:errorcluster, "Opt_Selector out"=w3588:refnum<class "Opt_Selector.lvclass">)  [unwired: 7 in]
            n1878 = local write "P8"(w3594) -> ()
            n1879 = local write "P9"(w3594) -> ()
            n1880 = local write "P10"(w3594) -> ()
            n1881 = local write "P11"(w3594) -> ()
            n1882 = local write "P12"(w3592) -> ()
            n1883 = local write "P13"(w3592) -> ()
            n1884 = local write "P14"(w3592) -> ()
            n1885 = local write "P15"(w3592) -> ()
          }
          frame 5 {
          }
        }
        n1886 = call "Write WPROT.vi"("error in (no error)"=w3492, "Opt_Selector.lvclass"=w3499, "Instrument in"=w3498) -> ("error out"=w3501:errorcluster, "Instrument out"=w3502:refnum<class "Instrument.lvclass">)  [unwired: 7 in]
        n1887 = property on="#Pol. Seq. Done" class="Slide (strict)"(error in=w3492, "Scale.Maximum"=w3493, "Scale.Minimum"=w3491) -> ()  [unwired: 1 in, 2 out]
        n1888 = call "Write Instrument.lvclass.vi"("error in (no error)"=w3501, "Instrument.lvclass"=w3502, "S4ACS_GUI in"=w3497) -> ("error out"=w3481:errorcluster, "S4ACS_GUI out"=w3482:refnum<class "S4GUI.lvclass">)  [unwired: 7 in]
        n1889 = call "Read Instrument.lvclass.vi"("error in (no error)"=w3481, "S4ACS_GUI in"=w3482) -> ("error out"=w3486:errorcluster, "Instrument.lvclass"=w3487:refnum<class "Instrument.lvclass">, "S4ACS_GUI out"=w3490:refnum<class "S4GUI.lvclass">)  [unwired: 7 in]
        n1890 = call "Read ASEL.vi"("error in (no error)"=w3486, "Instrument in"=w3487) -> ("error out"=w3476:errorcluster, "Opt_Selector.lvclass"=w3478:refnum<class "Opt_Selector.lvclass">, "Instrument out"=w3483:refnum<class "Instrument.lvclass">)  [unwired: 7 in]
        n1891 = call "Read name_pos.vi"("error in (no error)"=w3476, "Optics in"=w3478) -> ("error out"=w3475:errorcluster, "name_pos"=w3474:string, "Optics out"=w3477:refnum<class "Opt_Selector.lvclass">)  [unwired: 7 in]
        n1892 = call "Write ASEL.vi"("error in (no error)"=w3475, "Opt_Selector.lvclass"=w3477, "Instrument in"=w3483) -> ("error out"=w3484:errorcluster, "Instrument out"=w3488:refnum<class "Instrument.lvclass">)  [unwired: 7 in]
        n1893 = case shown="\"ON\"" w3474 {
          tunnel: w3484 -> [w3507 w3518]
          tunnel: [w3507 w3514] -> w3485
          tunnel: w3488 -> [w3506 w3519]
          tunnel: [w3506 w3515] -> w3489
          frame Default {
          }
          frame "ON" {
            n1894 = call "Read WPROT.vi"("error in (no error)"=w3518, "Instrument in"=w3519) -> ("error out"=w3510:errorcluster, "Opt_Selector.lvclass"=w3517:refnum<class "Opt_Selector.lvclass">, "Instrument out"=w3516:refnum<class "Instrument.lvclass">)  [unwired: 7 in]
            n1895 = call-dynamic "Read sequencia.vi"("error in (no error)"=w3510, "Opt_Selector in"=w3517) -> ("error out"=w3509:errorcluster, "sequencia"=w3513:u16, "Opt_Selector out"=w3512:refnum<class "Opt_Selector.lvclass">)  [unwired: 7 in]
            n1896 = case shown="0" w3513 {
              tunnel: w3512 -> [w3521 w3530]
              tunnel: [w3521 w3526] -> w3511
              tunnel: w3509 -> [w3520 w3529]
              tunnel: [w3520 w3524] -> w3508
              frame Default {
              }
              frame 0 {
                n1897 = call-dynamic "Write sequencia.vi"("error in (no error)"=w3529, "sequencia"=u16 1, "Opt_Selector in"=w3530) -> ("error out"=w3525:errorcluster, "Opt_Selector out"=w3527:refnum<class "Opt_Selector.lvclass">)  [unwired: 7 in]
                n1898 = local write "P0"(TRUE ("P0")) -> ()
                n1899 = call-dynamic "Write sequencia_ant.vi"("error in (no error)"=w3525, "sequencia_ant"=u16 1, "Opt_Selector in"=w3527) -> ("error out"=w3524:errorcluster, "Opt_Selector out"=w3526:refnum<class "Opt_Selector.lvclass">)  [unwired: 7 in]
              }
            }
            n1900 = call "Write WPROT.vi"("error in (no error)"=w3508, "Opt_Selector.lvclass"=w3511, "Instrument in"=w3516) -> ("error out"=w3514:errorcluster, "Instrument out"=w3515:refnum<class "Instrument.lvclass">)  [unwired: 7 in]
          }
        }
        n1901 = call "Write Instrument.lvclass.vi"("error in (no error)"=w3485, "Instrument.lvclass"=w3489, "S4ACS_GUI in"=w3490) -> ("error out"=w3480:errorcluster, "S4ACS_GUI out"=w3479:refnum<class "S4GUI.lvclass">)  [unwired: 7 in]
      }
      event "P0", "P1", "P2", "P3", "P4", "P5", "P6", "P7", "P8", "P9", "P10", "P11", "P12", "P13", "P14", "P15": Value Change {
        w3653 = u16 5 items=["All 16 positions", "First 8 positions", "First 4 positions", "0-3 + 8-11", "Clear", "Customized"] ("Select Positions")
        # "Garantir que, quando em POLARIMETRIA, pelo menos WP1 esteja selecionado."
        # "Salva tambem em \nSequencia_ant para\no caso de repeticao."
        n1902 = event-data() -> ()  [unwired: 1 in, 6 out]
        n1903 = call "Read Instrument.lvclass.vi"("error in (no error)"=w3635, "S4ACS_GUI in"=w3636) -> ("error out"=w3630:errorcluster, "Instrument.lvclass"=w3633:refnum<class "Instrument.lvclass">, "S4ACS_GUI out"=w3634:refnum<class "S4GUI.lvclass">)  [unwired: 7 in]
        n1904 = Build Array("P0", "P1", "P2", "P3", "P4", "P5", "P6", "P7", "P8", "P9", "P10", "P11", "P12", "P13", "P14", "P15") -> (w3621:bool[])
        n1905 = call "Read WPROT.vi"("error in (no error)"=w3630, "Instrument in"=w3633) -> ("error out"=w3629:errorcluster, "Opt_Selector.lvclass"=w3631:refnum<class "Opt_Selector.lvclass">, "Instrument out"=w3632:refnum<class "Instrument.lvclass">)  [unwired: 7 in]
        n1906 = local write "Select Positions"(w3653) -> ()
        n1907 = Boolean Array To Number(Boolean array=w3621) -> (number=w3637:u32)
